vi "Channel Enum to String.vi"(1 "OutputChannel":T1) -> (0 "format string":string)   [LabVIEW 2016, in "RP100.lvclass"]
uses:
  RP100.lvclass
  Typedefs/Output Channel--Enum.ctl
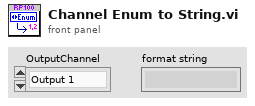
[diagram p1: front panel]
types:
  T1 = typedef "RP100.lvclass/Output Channel--Enum.ctl" = enum16{"Output 1", "Output 2"}
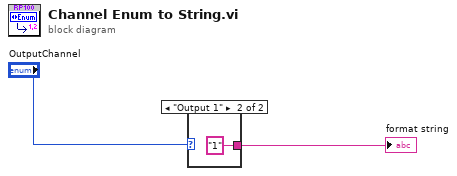
[diagram p0: block diagram]
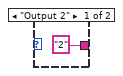
[diagram p2: hidden frame]
diagram:
  n1 = case shown="\"Output 1\"" "OutputChannel" {
    tunnel: ["2" ("format string") "1" ("format string")] -> w2
    frame "Output 2" {
    }
    frame "Output 1" {
    }
  }
  "format string" <- w2
